vi "New Default Style Object.vi"(8 "error in (no error)":errorcluster) -> (0 "error out":errorcluster, 3 "Style out":refnum<class "Style.lvclass">)   [LabVIEW 2020, in "Styles.lvlib" / "Style.lvclass"]
uses:
  Style.lvclass
  Style.lvclass/Style.ctl
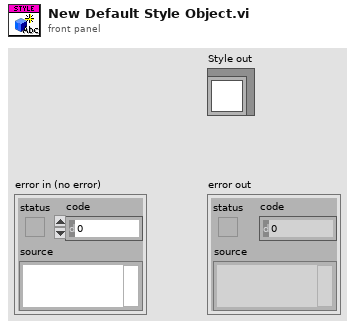
[diagram p1: front panel]
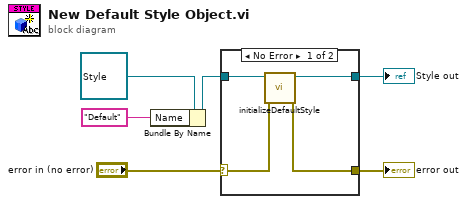
[diagram p0: block diagram]
diagram:
  n1 = Bundle By Name(cluster=refnum<class "Style.lvclass"> refnum ("Font in"), "Name"="Default" ("Style Name")) -> (w2:refnum<class "Style.lvclass">)
  n2 = case shown="No Error" "error in (no error)" {
    selector: "error in (no error)" -> [w8 w12]
    tunnel: w2 -> [w10 w11]
    tunnel: [w9 w11] -> w5
    tunnel: [w7 w12] -> w3
    frame No Error {
      n3 = call-dynamic "initializeDefaultStyle.vi"("error in (no error)"=w8, "Style in"=w10) -> ("error out"=w7:errorcluster, "Style out"=w9:refnum<class "Style.lvclass">)  [unwired: 8 in]
    }
    frame Error {
    }
  }
  "error out" <- w3
  "Style out" <- w5
